vi "SngJntArmSim_HasHitLowerLimit.vi"(11 "SingleJointArmSim":T1 {"GearBox"."Kt_NMPerAmp" format="%13.5p"; "GearBox"."Kv_RadPerSecPerVolt" format="%13.5p"; "GearBox"."R_Ohms" format="%13.5p"; "GearBox"."FreeSpeed_RadPerSec" format="%13.5p"; "GearBox"."FreeCurrent_Amps" format="%13.5p"; "GearBox"."StallCurrent_Amps" format="%13.5p"; "GearBox"."StallTorque_NM" format="%13.5p"; "GearBox"."nominalVoltage_Volts" format="%13.5p"}) -> (3 "AtLowLimit":bool)   [LabVIEW 2019, in "Trajectory_Library.lvlib"]
doc: "Creates a new LINEAR SYSTEM data cluster with the specified values. \n\n\nInputs: \n - XXX -- XXX.\n\nOutputs:\n - XXX -- XXX."
uses:
  Trajectory_Library.lvlib
  SINGLE_JOINT_ARM_SIM.ctl
  LINEAR_SYSTEM_SIM.ctl
  LINEAR_SYSTEM.ctl
  <vilib>/Analysis/Matrix/Datatypes/RealMatrix.ctl
  DCMOTOR.CTL
  <vilib>/Analysis/Matrix/NI_Matrix.lvlib
panel:
  # "<States, 1>"
  # "<Outputs, 1>"
  # "<Inputs, 1>"
  # "<Outputs, 1>"
  # "<States,States>"
  # "<States,Inputs>"
  # "<Outputs,States>"
  # "<Outputs,Inputs>"
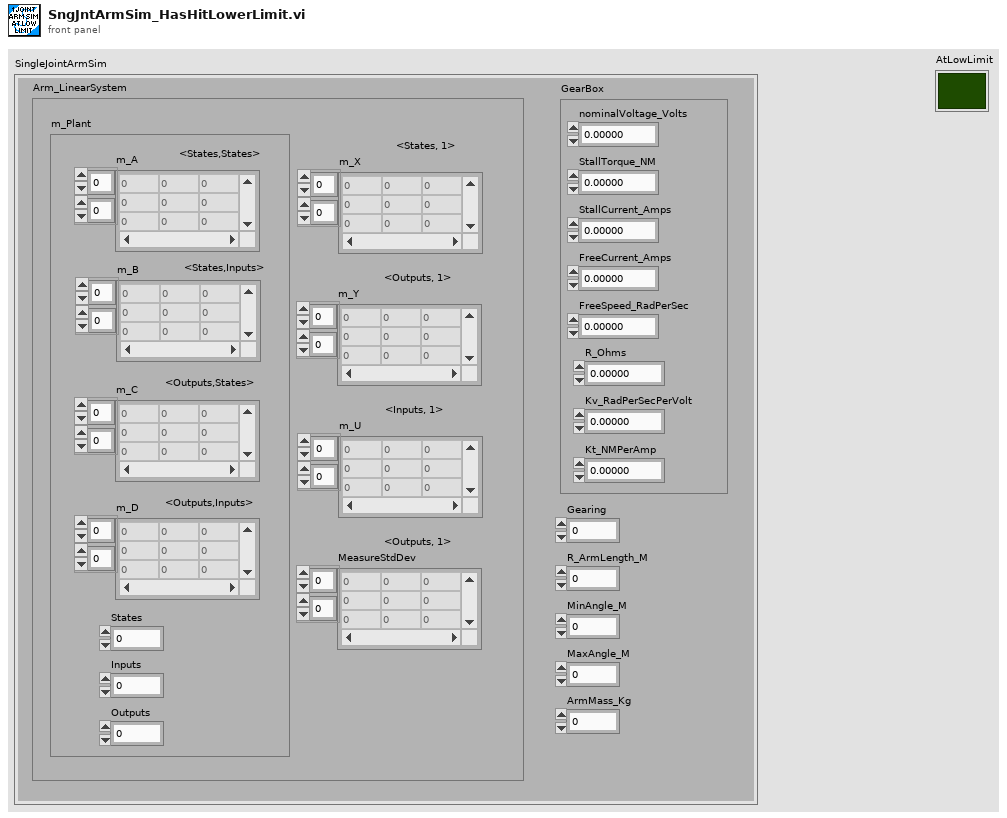
[diagram p1: front panel]
types:
  T1 = typedef "Trajectory_Library.lvlib/SINGLE_JOINT_ARM_SIM.ctl" = cluster{"Arm_LinearSystem":T2, "GearBox":T5, "Gearing":dbl, "R_ArmLength_M":dbl, "MinAngle_M":dbl, "MaxAngle_M":dbl, "ArmMass_Kg":dbl}
  T2 = typedef "Trajectory_Library.lvlib/LINEAR_SYSTEM_SIM.ctl" = cluster{"m_Plant":T3, "m_X":T4, "m_Y":T4, "m_U":T4, "MeasureStdDev":T4}
  T3 = typedef "Trajectory_Library.lvlib/LINEAR_SYSTEM.ctl" = cluster{"m_A":T4, "m_B":T4, "m_C":T4, "m_D":T4, "States":i32, "Inputs":i32, "Outputs":i32}
  T4 = typedef "NI_Matrix.lvlib/RealMatrix.ctl" = dbl[][]
  T5 = typedef "Trajectory_Library.lvlib/DCMOTOR.CTL" = cluster{"nominalVoltage_Volts":dbl, "StallTorque_NM":dbl, "StallCurrent_Amps":dbl, "FreeCurrent_Amps":dbl, "FreeSpeed_RadPerSec":dbl, "R_Ohms":dbl, "Kv_RadPerSecPerVolt":dbl, "Kt_NMPerAmp":dbl}
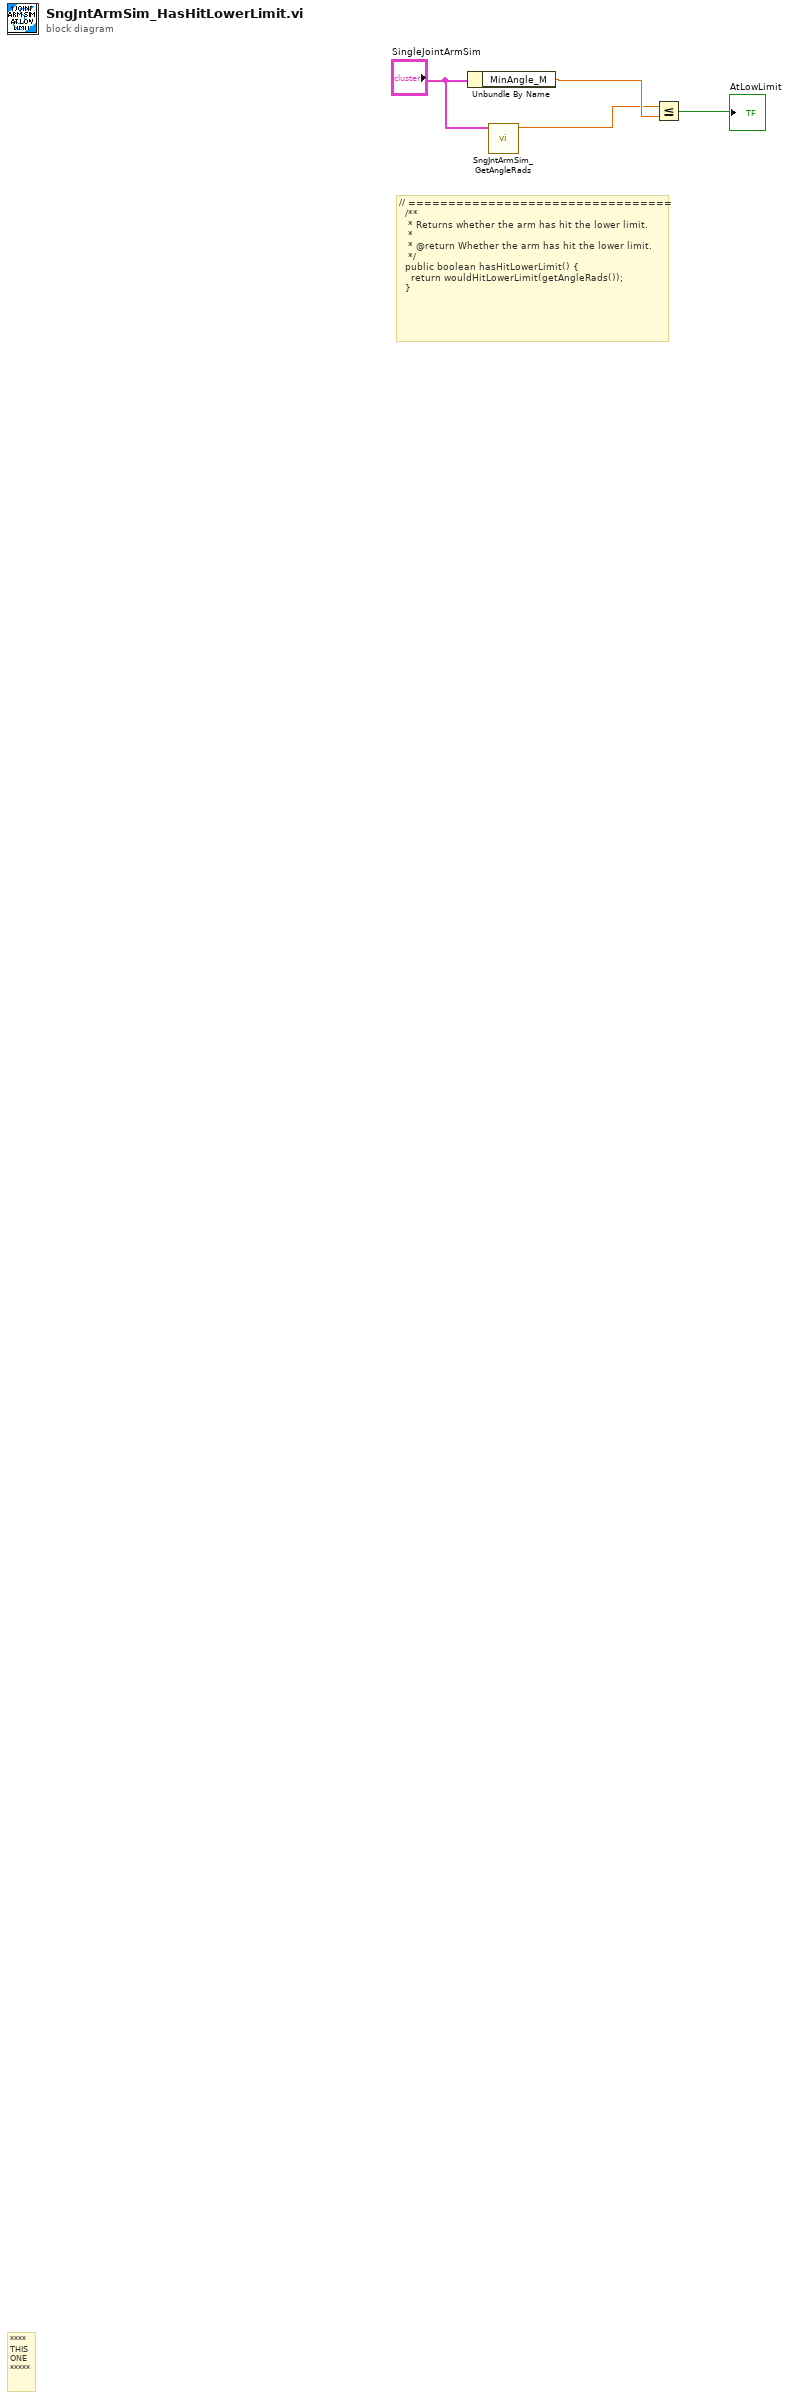
[diagram p0: block diagram]
diagram:
  # "// =================================\n  /**\n   * Returns whether the arm has hit the lower limit.\n   *\n   * @return Whether the arm has hit the lower limit.\n   */\n  public boolean hasHitLowerLimit() {\n    return wouldHitLowerLimit(getAngleRads());\n  }"
  # "****\nTHIS\nONE\n*****"
  n1 = Unbundle By Name("SingleJointArmSim") -> ("MinAngle_M"=w4:dbl)
  n2 = call "SngJntArmSim_GetAngleRads.vi"("SingleJointArmSim"="SingleJointArmSim") -> ("ArmAngle_Rad"=w1:dbl)  [unwired: 10 in]
  n3 = Less Or Equal?(x=w1, y=w4) -> (x <= y?=→"AtLowLimit":bool)
